vi "Display Info.vi"(7 "Layout ref":refnum<vi>, 8 "error in (no error)":errorcluster, 9 "Modify (F) /Add [T]":bool, 10 "Names in use":string[](array[string])=["PB", "Feet"], 11 "Pulseblaster in":refnum<class "Slave_Pulseblaster.lvclass">=refnum) -> (0 "error out":errorcluster, 1 "Names in use out":string[](array[string]), 2 "Changes Made?":bool, 3 "Pulseblaster out":refnum<class "Slave_Pulseblaster.lvclass">)   [LabVIEW 2013, in "Slave_Pulseblaster.lvclass"]
uses:
  Slave_Pulseblaster.lvclass
  ColumnVIs/DigitalCol/DigitalCol.lvclass
  ColumnVIs/Column/Column.lvclass
  TypeDefs/DigitalColumnAppearCluster.ctl
panel:
  in  "Trig.\nLine":i32=23 max=256 step=1
  in  "Digital Columns":T1[](array[typedef])=[{"Column Name"="", "Width"=15, "Bkgd"=[1985280, 6618880, 14090026], "Text"=[16448250, 0, 0]}, {"Column Name"="", "Width"=15, "Bkgd"=[1985280, 6618880, 14090026], "Text"=[16448250, 0, 0]}, {"Column Name"="", "Width"=15, "Bkgd"=[1985280, 6618880, 14090026], "Text"=[16448250, 0, 0]}, {"Column Name"="", "Width"=15, "Bkgd"=[1985280, 6618880, 14090026], "Text"=[16448250, 0, 0]}, {"Column Name"="", "Width"=15, "Bkgd"=[1985280, 6618880, 14090026], "Text"=[16448250, 0, 0]}, {"Column Name"="", "Width"=15, "Bkgd"=[1985280, 6618880, 14090026], "Text"=[16448250, 0, 0]}, {"Column Name"="", "Width"=15, "Bkgd"=[1985280, 6618880, 14090026], "Text"=[16448250, 0, 0]}, {"Column Name"="", "Width"=15, "Bkgd"=[1985280, 6618880, 14090026], "Text"=[16448250, 0, 0]}, {"Column Name"="", "Width"=15, "Bkgd"=[1985280, 6618880, 14090026], "Text"=[16448250, 0, 0]}, {"Column Name"="", "Width"=15, "Bkgd"=[1985280, 6618880, 14090026], "Text"=[16448250, 0, 0]}, {"Column Name"="", "Width"=15, "Bkgd"=[1985280, 6618880, 14090026], "Text"=[16448250, 0, 0]}, {"Column Name"="", "Width"=15, "Bkgd"=[1985280, 6618880, 14090026], "Text"=[16448250, 0, 0]}, {"Column Name"="", "Width"=15, "Bkgd"=[1985280, 6618880, 14090026], "Text"=[16448250, 0, 0]}, {"Column Name"="", "Width"=15, "Bkgd"=[1985280, 6618880, 14090026], "Text"=[16448250, 0, 0]}, {"Column Name"="", "Width"=15, "Bkgd"=[1985280, 6618880, 14090026], "Text"=[16448250, 0, 0]}, {"Column Name"="", "Width"=15, "Bkgd"=[1985280, 6618880, 14090026], "Text"=[16448250, 0, 0]}, {"Column Name"="", "Width"=15, "Bkgd"=[1985280, 6618880, 14090026], "Text"=[16448250, 0, 0]}, {"Column Name"="", "Width"=15, "Bkgd"=[1985280, 6618880, 14090026], "Text"=[16448250, 0, 0]}, {"Column Name"="", "Width"=15, "Bkgd"=[1985280, 6618880, 14090026], "Text"=[16448250, 0, 0]}, {"Column Name"="", "Width"=15, "Bkgd"=[1985280, 6618880, 14090026], "Text"=[16448250, 0, 0]}, {"Column Name"="", "Width"=15, "Bkgd"=[1985280, 6618880, 14090026], "Text"=[16448250, 0, 0]}, {"Column Name"="", "Width"=15, "Bkgd"=[1985280, 6618880, 14090026], "Text"=[16448250, 0, 0]}, {"Column Name"="", "Width"=15, "Bkgd"=[1985280, 6618880, 14090026], "Text"=[16448250, 0, 0]}, {"Column Name"="", "Width"=15, "Bkgd"=[1985280, 6618880, 14090026], "Text"=[16448250, 0, 0]}]
  in  "Set All Digitals":T1={"Column Name"="", "Width"=15, "Bkgd"=[1985280, 6618880, 14090026], "Text"=[16448250, 0, 0]}
  in  "Board Num.":i32=1 max=256 step=1
  in  "SpinAPI Path":path=path "C:/SpinCore/SpinAPI/dll/spinapi.dll"
  out "Digital Cols":refnum<class "Column.lvclass">[](array[class])
  in  "Cancel":bool
  in  "Done":bool
  in  "Device Description":string="Othe rfeet"
  in  "Name":string="Feet"
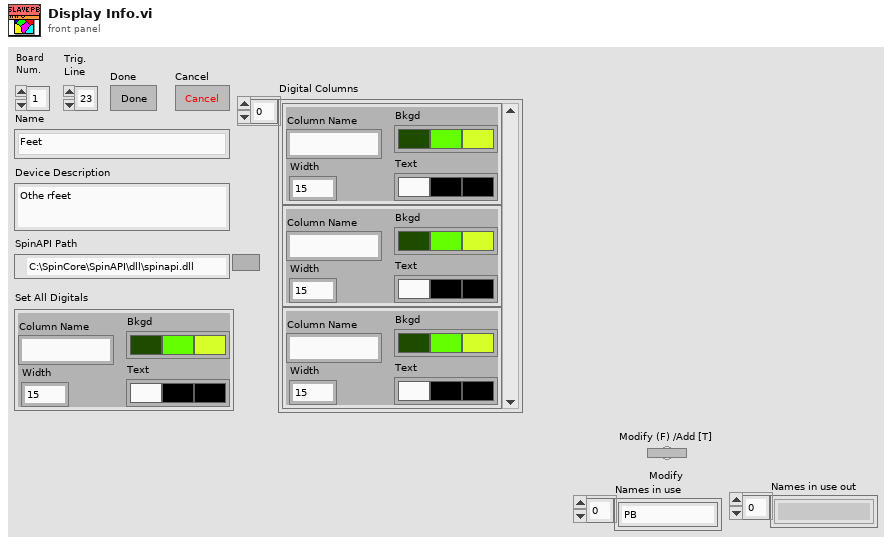
[diagram p1: front panel]
types:
  T1 = typedef "DigitalColumnAppearCluster.ctl" = cluster{"Column Name":string, "Width":u32, "Bkgd":u32[], "Text":u32[]}
  T2 = typedef "ColumnAppearCluster.ctl" = cluster{"Column Name":string, "Width":u32, "Bkgd":u32[], "Text":u32[]}
  T3 = cluster{"Column Name":bool, "Width":bool, "Bkgd":bool[], "Text":bool[]}[]
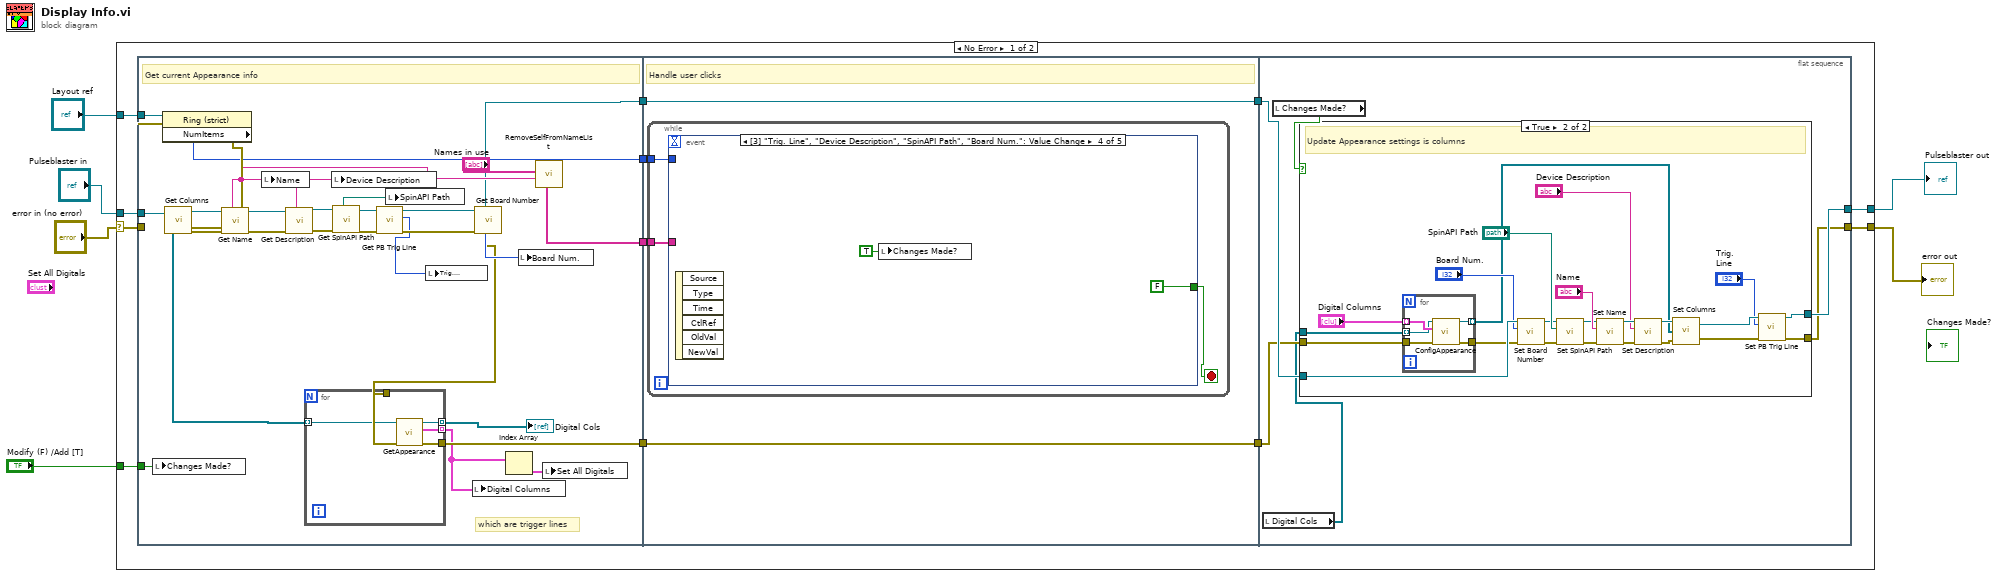
[diagram p0: block diagram]
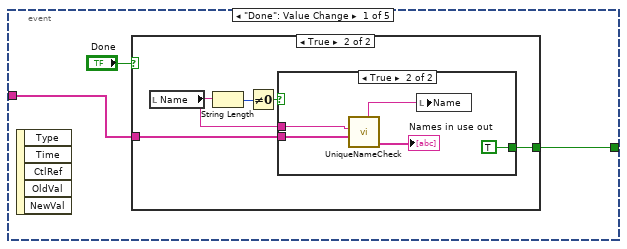
[diagram p2: hidden frame]
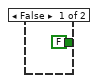
[diagram p3: hidden frame]
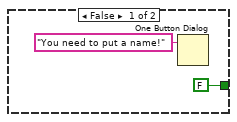
[diagram p4: hidden frame]
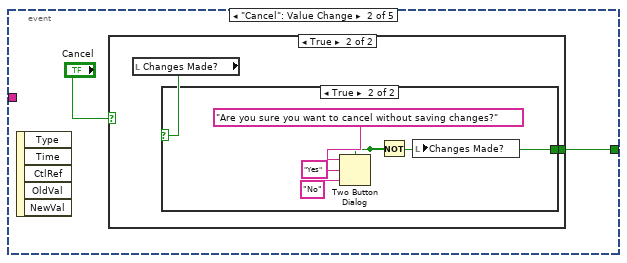
[diagram p5: hidden frame]
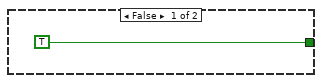
[diagram p7: hidden frame]
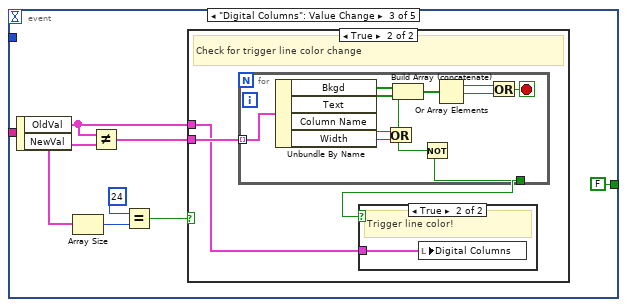
[diagram p8: hidden frame]
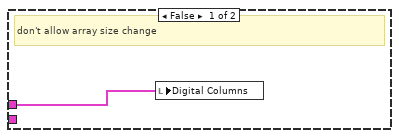
[diagram p9: hidden frame]
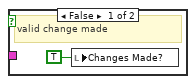
[diagram p10: hidden frame]
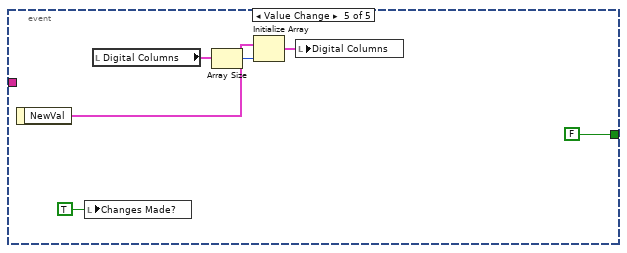
[diagram p11: hidden frame]
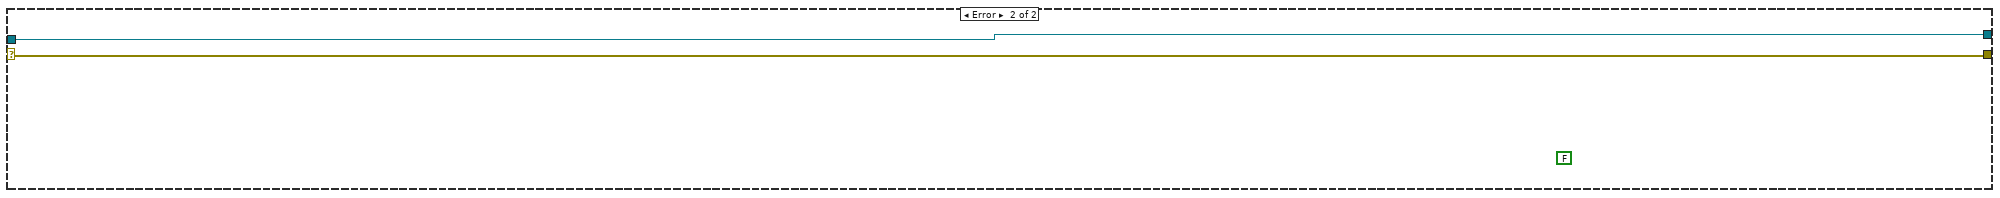
[diagram p13: hidden frame]
diagram:
  n1 = case shown="No Error" "error in (no error)" {
    selector: "error in (no error)" -> [w11 w155]
    tunnel: [w13 w156] -> w5
    tunnel: "Pulseblaster in" -> [w18 w156]
    tunnel: [w12 w155] -> w3
    tunnel: "Layout ref" -> [w10 _]
    tunnel: "Modify (F) /Add [T]" -> [w8 _]
    frame No Error {
      n2 = flat-sequence {
        tunnel: w18 -> [w46]
        tunnel: [w30] -> w17
        tunnel: [w42] -> w15
        tunnel: w11 -> [w39]
        tunnel: w10 -> [w40]
        tunnel: [w37] -> w9
        tunnel: w8 -> [w36]
        tunnel: [w33] -> w7
        tunnel: w17 -> [w57]
        tunnel: [w57] -> w16
        tunnel: w15 -> [w56]
        tunnel: [w56] -> w14
        tunnel: w9 -> [w55]
        tunnel: w7 -> [w54]
        tunnel: w16 -> [w123]
        tunnel: w14 -> [w120]
        tunnel: [w122] -> w13
        tunnel: [w121] -> w12
        frame #0 {
          # "which are trigger lines"
          # "Get current Appearance info"
          n3 = local write "Changes Made?"(w36) -> ()
          n4 = property class="Ring (strict)"(reference=w40, error in=w39) -> (error out=w38:errorcluster, "NumItems"=w37:u32)  [unwired: 1 out]
          n5 = call-dynamic "Get Columns.vi"("Device in"=w46, "error in (no error)"=w38) -> ("Device out"=w44:refnum<class "Slave_Pulseblaster.lvclass">, "Columns"=w27:refnum<class "Column.lvclass">[], "error out"=w43:errorcluster)
          n6 = call-dynamic "Get Name.vi"("error in (no error)"=w43, "Device in"=w44) -> ("error out"=w45:errorcluster, "Name"=w34:string, "Device out"=w48:refnum<class "Slave_Pulseblaster.lvclass">)  [unwired: 7 in]
          n7 = local write "Name"(w34) -> ()
          n8 = call-dynamic "Get Description.vi"("error in (no error)"=w45, "Device in"=w48) -> ("error out"=w31:errorcluster, "Device Description"=w47:string, "Device out"=w32:refnum<class "Slave_Pulseblaster.lvclass">)  [unwired: 7 in]
          n9 = local write "Device Description"(w47) -> ()
          n10 = call-dynamic "Get SpinAPI Path.vi"("error in (no error)"=w31, "Pulseblaster in"=w32) -> ("error out"=w22:errorcluster, "SpinAPI Path"=w28:path, "Pulseblaster out"=w23:refnum<class "Slave_Pulseblaster.lvclass">)  [unwired: 7 in]
          n11 = call-dynamic "Get PB Trig Line.vi"("error in (no error)"=w22, "Device in"=w23) -> ("error out"=w20:errorcluster, "PB Trigger Line"=w19:u16, "Device out"=w21:refnum<class "Slave_Pulseblaster.lvclass">)  [unwired: 7 in]
          n12 = local write "SpinAPI Path"(w28) -> ()
          n13 = local write "Trig.\nLine"(w19) -> ()
          n14 = call-dynamic "Get Board Number.vi"("error in (no error)"=w20, "Pulseblaster in"=w21) -> ("error out"=w26:errorcluster, "Board Number"=w29:i32, "Pulseblaster out"=w30:refnum<class "Slave_Pulseblaster.lvclass">)  [unwired: 7 in]
          n15 = for {
            tunnel: w27 -> [w49] mode=indexing
            tunnel: [w53] -> w24 mode=indexing
            tunnel: [w52] -> w42
            tunnel: w26 -> [w51]
            tunnel: [w50] -> w25 mode=indexing
            n16 = call "GetAppearance.vi"("error in (no error)"=w51, "Column in"=w49) -> ("error out"=w52:errorcluster, "Column Appearance"=w53:T2, "Column out"=w50:refnum<class "Column.lvclass">)  [unwired: 7 in]
          }
          "Digital Cols" <- w25
          n17 = local write "Digital Columns"(w24) -> ()
          n18 = Index Array(array=w24) -> (element=w41:T2)  [unwired: 1 in]
          n19 = local write "Board Num."(w29) -> ()
          n20 = call "RemoveSelfFromNameList.vi"("self Name"=w34, "Names in use"="Names in use") -> ("Reserved Names"=w33:string[])  [unwired: 9 in]
          n21 = local write "Set All Digitals"(w41) -> ()
        }
        frame #1 {
          # "Handle user clicks"
          n22 = while {
            tunnel: w55 -> [w59]
            tunnel: w54 -> [w58]
            stop <- w60 stop-if-true
            n23 = event shown="[3] \"Trig. Line\", \"Device Description\", \"SpinAPI Path\", \"Board Num.\": Value Change" {
              selector: _ -> [_ _ _ _ _]
              dyn-events: _ -> [_ _ _ _ _]
              timeout: _ -> [_ _ _ _ _]
              tunnel: [w62 w78 FALSE ("T button?") FALSE ("T button?") FALSE ("T button?")] -> w60
              tunnel: w59 -> [_ _ _ _ _]
              tunnel: w58 -> [w61 _ _ _ _]
              event "Done": Value Change {
                n24 = event-data() -> ()  [unwired: 1 in, 5 out]
                n25 = case shown="True" "Done" {
                  tunnel: [FALSE w67] -> w62
                  tunnel: w61 -> [_ w65]
                  frame False {
                  }
                  frame True {
                    n26 = local read "Name"() -> (w66:string)
                    n27 = String Length(string=w66) -> (length=w69:i32)
                    n28 = Not Equal To 0?(x=w69) -> (x != 0?=w68:bool)
                    n29 = case shown="True" w68 {
                      tunnel: [FALSE TRUE] -> w67
                      tunnel: w66 -> [_ w75]
                      tunnel: w65 -> [_ w73]
                      frame False {
                        n30 = One Button Dialog(message="You need to put a name!") -> ()  [unwired: 1 in, 1 out]
                      }
                      frame True {
                        n31 = call "UniqueNameCheck.vi"("Names in use"=w73, "Device Name"=w75) -> ("Names in use out"=→"Names in use out":string[], "Unique name"=w74:string)  [unwired: 8 in]
                        n32 = local write "Name"(w74) -> ()
                      }
                    }
                  }
                }
              }
              event "Cancel": Value Change {
                n33 = event-data() -> ()  [unwired: 1 in, 5 out]
                n34 = case shown="True" "Cancel" {
                  selector: "Cancel" -> [w79 _]
                  tunnel: [w79 w81] -> w78
                  frame False {
                  }
                  frame True {
                    n35 = local read "Changes Made?"() -> (w80:bool)
                    n36 = case shown="True" w80 {
                      tunnel: [TRUE w84] -> w81
                      frame False {
                      }
                      frame True {
                        n37 = Two Button Dialog(message="Are you sure you want to cancel without saving changes?", 1:"No", 2:"Yes") -> (T button?=w84:bool)
                        n38 = Not(x=w84) -> (.not. x?=w83:bool)
                        n39 = local write "Changes Made?"(w83) -> ()
                      }
                    }
                  }
                }
              }
              event "Digital Columns": Value Change {
                n40 = event-data() -> ("OldVal"=w88:T1[], "NewVal"=w90:T1[])  [unwired: 1 in]
                n41 = Array Size(array=w90) -> (size(s)=w93:i32)
                n42 = Not Equal?(x=w88, y=w90) -> (x != y?=w89:T3)
                n43 = Equal?(x=24 ("y"), y=w93) -> (x = y?=w94:bool)
                n44 = case shown="True" w94 {
                  tunnel: w88 -> [w95 w96]
                  tunnel: w89 -> [_ w98]
                  frame False {
                    # "don't allow array size change"
                    n45 = local write "Digital Columns"(w95) -> ()
                  }
                  frame True {
                    # "Check for trigger line color change"
                    n46 = for {
                      tunnel: w98 -> [w110] mode=indexing
                      tunnel: [w101] -> w97
                      stop <- w106 stop-if-true
                      n47 = Unbundle By Name(w110) -> ("Bkgd"=w109:bool[], "Text"=w108:bool[], "Column Name"=w104:bool, "Width"=w103:bool)
                      n48 = Or(x=w104, y=w103) -> (x .or. y?=w102:bool)
                      n49 = Build Array (concatenate)(w109, w108) -> (w107:bool[])
                      n50 = Not(x=w102) -> (.not. x?=w101:bool)
                      n51 = Or Array Elements(Boolean array=w107) -> (logical OR=w105:bool)
                      n52 = Or(x=w105, y=w102) -> (x .or. y?=w106:bool)
                    }
                    n53 = case shown="True" w97 {
                      tunnel: w96 -> [_ w100]
                      frame False {
                        # "valid change made"
                        n54 = local write "Changes Made?"(TRUE ("Changes Made?")) -> ()
                      }
                      frame True {
                        # "Trigger line color!"
                        n55 = local write "Digital Columns"(w100) -> ()
                      }
                    }
                  }
                }
              }
              event "Trig.\nLine", "Device Description", "SpinAPI Path", "Board Num.": Value Change {
                n56 = event-data() -> ()  [unwired: 1 in, 6 out]
                n57 = local write "Changes Made?"(TRUE) -> ()
              }
              event Value Change {
                n58 = event-data() -> ("NewVal"=w116:T1)  [unwired: 1 in]
                n59 = local write "Changes Made?"(TRUE) -> ()
                n60 = local read "Digital Columns"() -> (w114:T1[])
                n61 = Array Size(array=w114) -> (size(s)=w113:i32)
                n62 = Initialize Array(w116, w113) -> (w115:T1[])
                n63 = local write "Digital Columns"(w115) -> ()
              }
            }
          }
        }
        frame #2 {
          n64 = local read "Digital Cols"() -> (w119:refnum<class "Column.lvclass">[])
          n65 = local read "Changes Made?"() -> (w124:bool)
          n66 = case shown="True" w124 {
            tunnel: w123 -> [w126 w138]
            tunnel: [w125 w128] -> w121
            tunnel: [w126 w129] -> w122
            tunnel: w120 -> [w125 w144]
            tunnel: w119 -> [_ w143]
            frame False {
            }
            frame True {
              # "Update Appearance settings is columns"
              n67 = for {
                tunnel: "Digital Columns" -> [w154] mode=indexing
                tunnel: [w153] -> w133 mode=indexing
                tunnel: [w152] -> w132
                tunnel: w143 -> [w151] mode=indexing
                tunnel: w144 -> [w150]
                n68 = call "ConfigAppearance.vi"("error in (no error)"=w150, "Column Appearance"=w154, "Column in"=w151) -> ("error out"=w152:errorcluster, "Column out"=w153:refnum<class "Column.lvclass">)  [unwired: 7 in]
              }
              n69 = call-dynamic "Set Board Number.vi"("error in (no error)"=w132, "Board Number"="Board Num.", "Pulseblaster in"=w138) -> ("error out"=w139:errorcluster, "Pulseblaster out"=w137:refnum<class "Slave_Pulseblaster.lvclass">)  [unwired: 7 in]
              n70 = call-dynamic "Set SpinAPI Path.vi"("error in (no error)"=w139, "SpinAPI Path"="SpinAPI Path", "Pulseblaster in"=w137) -> ("error out"=w140:errorcluster, "Pulseblaster out"=w136:refnum<class "Slave_Pulseblaster.lvclass">)  [unwired: 7 in]
              n71 = call-dynamic "Set Name.vi"("error in (no error)"=w140, "Name"="Name", "Device in"=w136) -> ("error out"=w149:errorcluster, "Device out"=w148:refnum<class "Slave_Pulseblaster.lvclass">)  [unwired: 7 in]
              n72 = call-dynamic "Set Description.vi"("error in (no error)"=w149, "Device Description"="Device Description", "Device in"=w148) -> ("error out"=w142:errorcluster, "Device out"=w147:refnum<class "Slave_Pulseblaster.lvclass">)  [unwired: 7 in]
              n73 = call-dynamic "Set Columns.vi"("error in (no error)"=w142, "Columns in"=w133, "Pulseblaster in"=w147) -> ("error out"=w131:errorcluster, "Pulseblaster out"=w130:refnum<class "Slave_Pulseblaster.lvclass">)  [unwired: 1 in]
              n74 = call-dynamic "Set PB Trig Line.vi"("error in (no error)"=w131, "PB Trigger Line"="Trig.\nLine", "Device in"=w130) -> ("error out"=w128:errorcluster, "Device out"=w129:refnum<class "Slave_Pulseblaster.lvclass">)  [unwired: 7 in]
            }
          }
        }
      }
    }
    frame Error {
      (unwired) FALSE
    }
  }
  "error out" <- w3
  "Pulseblaster out" <- w5
